vi "Parse Response Message.vi"(11 "message":string) -> (3 "response":T1 {"header"."response code" items=["NoError"=0, "FormErr"=1, "ServFail"=2, "NXDomain"=3, "NotImp"=4, "Refused"=5, "YXDomain"=6, "YXRRSet"=7, "NXRRSet"=8, "NotAuth"=9, "NotZone"=10, "DSOTYPENI"=11, "BADVERS/BADSIG"=16, "BADKEY"=17, "BADTIME"=18, "BADMODE"=19, "BADNAME"=20, "BADALG"=21, "BADTRUNC"=22, "BADCOOKIE"=23]; "header"."opcode" items=["Query"=0, "IQuery"=1, "Status"=2, "Notify"=4, "Update"=5, "DSO"=6]; "additional records"."class" items=["IN"=1, "CH"=3, "HS"=4]; "additional records"."type" items=["A"=1, "NS"=2, "MD"=3, "MF"=4, "CNAME"=5, "SOA"=6, "MB"=7, "MG"=8, "MR"=9, "NULL"=10, "WKS"=11, "PTR"=12, "HINFO"=13, "MINFO"=14, "MX"=15, "TXT"=16, "RP"=17, "AFSDB"=18, "X25"=19, "ISDN"=20, "RT"=21, "NSAP"=22, "NSAP-PTR"=23, "SIG"=24, "KEY"=25, "PX"=26, "GPOS"=27, "AAAA"=28, "LOC"=29, "NXT"=30, "EID"=31, "NIMLOC"=32, "SRV"=33, "ATMA"=34, "NAPTR"=35, "KX"=36, "CERT"=37, "A6"=38, "DNAME"=39, "SINK"=40, "OPT"=41, "APL"=42, "DS"=43, "SSHFP"=44, "IPSECKEY"=45, "RRSIG"=46, "NSEC"=47, "DNSKEY"=48, "DHCID"=49, "NSEC3"=50, "NSEC3PARAM"=51, "TLSA"=52, "SMIMEA"=53, "HIP"=55, "NINFO"=56, "RKEY"=57, "TALINK"=58, "CDS"=59, "CDNSKEY"=60, "OPENPGPKEY"=61, "CSYNC"=62, "ZONEMD"=63, "SVCB"=64, "HTTPS"=65, "SPF"=99, "UINFO"=100, "UID"=101, "GID"=102, "UNSPEC"=103, "NID"=104, "L32"=105, "L64"=106, "LP"=107, "EUI48"=108, "EUI64"=109, "URI"=256, "CAA"=257, "AVC"=258, "DOA"=259, "AMTRELAY"=260, "TA"=32768, "DLV"=32769]; "authority records"."class" items=["IN"=1, "CH"=3, "HS"=4]; "authority records"."type" items=["A"=1, "NS"=2, "MD"=3, "MF"=4, "CNAME"=5, "SOA"=6, "MB"=7, "MG"=8, "MR"=9, "NULL"=10, "WKS"=11, "PTR"=12, "HINFO"=13, "MINFO"=14, "MX"=15, "TXT"=16, "RP"=17, "AFSDB"=18, "X25"=19, "ISDN"=20, "RT"=21, "NSAP"=22, "NSAP-PTR"=23, "SIG"=24, "KEY"=25, "PX"=26, "GPOS"=27, "AAAA"=28, "LOC"=29, "NXT"=30, "EID"=31, "NIMLOC"=32, "SRV"=33, "ATMA"=34, "NAPTR"=35, "KX"=36, "CERT"=37, "A6"=38, "DNAME"=39, "SINK"=40, "OPT"=41, "APL"=42, "DS"=43, "SSHFP"=44, "IPSECKEY"=45, "RRSIG"=46, "NSEC"=47, "DNSKEY"=48, "DHCID"=49, "NSEC3"=50, "NSEC3PARAM"=51, "TLSA"=52, "SMIMEA"=53, "HIP"=55, "NINFO"=56, "RKEY"=57, "TALINK"=58, "CDS"=59, "CDNSKEY"=60, "OPENPGPKEY"=61, "CSYNC"=62, "ZONEMD"=63, "SVCB"=64, "HTTPS"=65, "SPF"=99, "UINFO"=100, "UID"=101, "GID"=102, "UNSPEC"=103, "NID"=104, "L32"=105, "L64"=106, "LP"=107, "EUI48"=108, "EUI64"=109, "URI"=256, "CAA"=257, "AVC"=258, "DOA"=259, "AMTRELAY"=260, "TA"=32768, "DLV"=32769]; "answers"."class" items=["IN"=1, "CH"=3, "HS"=4]; "answers"."type" items=["A"=1, "NS"=2, "MD"=3, "MF"=4, "CNAME"=5, "SOA"=6, "MB"=7, "MG"=8, "MR"=9, "NULL"=10, "WKS"=11, "PTR"=12, "HINFO"=13, "MINFO"=14, "MX"=15, "TXT"=16, "RP"=17, "AFSDB"=18, "X25"=19, "ISDN"=20, "RT"=21, "NSAP"=22, "NSAP-PTR"=23, "SIG"=24, "KEY"=25, "PX"=26, "GPOS"=27, "AAAA"=28, "LOC"=29, "NXT"=30, "EID"=31, "NIMLOC"=32, "SRV"=33, "ATMA"=34, "NAPTR"=35, "KX"=36, "CERT"=37, "A6"=38, "DNAME"=39, "SINK"=40, "OPT"=41, "APL"=42, "DS"=43, "SSHFP"=44, "IPSECKEY"=45, "RRSIG"=46, "NSEC"=47, "DNSKEY"=48, "DHCID"=49, "NSEC3"=50, "NSEC3PARAM"=51, "TLSA"=52, "SMIMEA"=53, "HIP"=55, "NINFO"=56, "RKEY"=57, "TALINK"=58, "CDS"=59, "CDNSKEY"=60, "OPENPGPKEY"=61, "CSYNC"=62, "ZONEMD"=63, "SVCB"=64, "HTTPS"=65, "SPF"=99, "UINFO"=100, "UID"=101, "GID"=102, "UNSPEC"=103, "NID"=104, "L32"=105, "L64"=106, "LP"=107, "EUI48"=108, "EUI64"=109, "URI"=256, "CAA"=257, "AVC"=258, "DOA"=259, "AMTRELAY"=260, "TA"=32768, "DLV"=32769]})   [LabVIEW 2015, in "PL DNS Client.lvlib"]
doc: "Parses DNS response <b>message</b>."
uses:
  PL DNS Client.lvlib
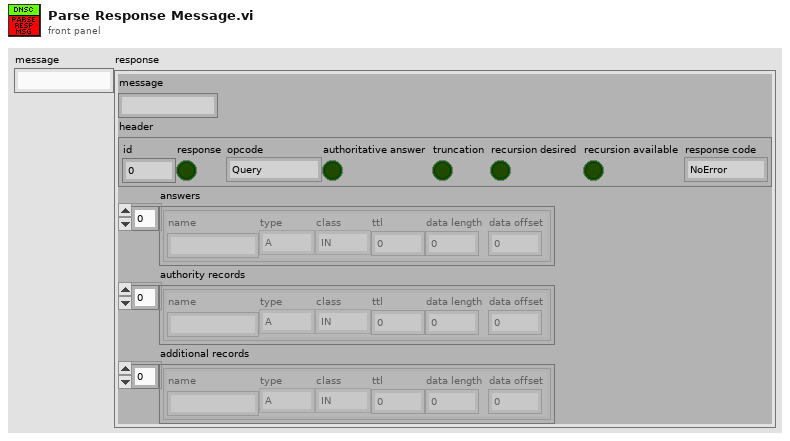
[diagram p1: front panel]
types:
  T1 = cluster{"message":string, "header":cluster{"id":u16, "response":bool, "opcode":u8, "authoritative answer":bool, "truncation":bool, "recursion desired":bool, "recursion available":bool, "response code":u16}, "answers":cluster{"name":string, "type":u16, "class":u16, "ttl":u32, "data length":u16, "data offset":u16}[], "authority records":cluster{"name":string, "type":u16, "class":u16, "ttl":u32, "data length":u16, "data offset":u16}[], "additional records":cluster{"name":string, "type":u16, "class":u16, "ttl":u32, "data length":u16, "data offset":u16}[]}
  T2 = cluster{"name":string, "type":u16, "class":u16, "ttl":u32, "data length":u16, "data offset":u16}
  T3 = cluster{cluster{"name":string, "type":u16, "class":u16, "ttl":u32, "data length":u16, "data offset":u16}[]}
  T4 = cluster{"name":string, "type":u16, "class":u16, "ttl":u32, "data length":u16, "data offset":u16}[]
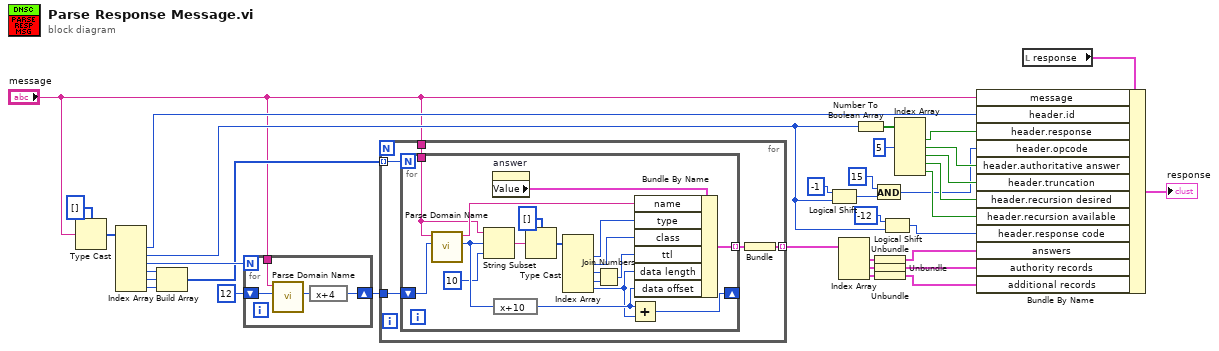
[diagram p0: block diagram]
diagram:
  n1 = Type Cast(type=u16[] [] ("array"), x="message") -> (*(type *) &x=w33:u16[])
  n2 = Index Array(array=w33) -> (element #1=w13:u16, element #2=w2:u16, element #3=w32:u16, element #4=w31:u16, element #5=w29:u16, element #6=w30:u16)  [unwired: 6 in]
  n3 = Build Array(w31, w29, w30) -> (w28:u16[])
  n4 = for {
    N: w32 -> [_]
    shift-right: [w36] -> w27
    shift-left: u16 12 -> [w38]
    tunnel: "message" -> [w35]
    n5 = call "Parse Domain Name.vi"("offset"=w38, "message"=w35) -> ("offset past domain name"=w37:u16)  [unwired: 8 in, 1 out]
    n6 = expression code="x+4"(w37) -> (w36:u16)
  }
  n7 = for {
    tunnel: w27 -> [w43]
    tunnel: "message" -> [w42]
    tunnel: w28 -> [w41] mode=indexing
    tunnel: [w39] -> w25 mode=indexing
    n8 = for {
      N: w41 -> [_]
      tunnel: w42 -> [w46]
      shift-right: [w60] -> _
      shift-left: w43 -> [w58]
      tunnel: [w61] -> w40 mode=indexing
      n9 = call "Parse Domain Name.vi"("offset"=w58, "message"=w46) -> ("offset past domain name"=w45:u16, "domain name"=w55:string)  [unwired: 8 in]
      n10 = String Subset(string=w46, offset (0)=w45, length (rest)=10 ("length")) -> (substring=w53:string)
      n11 = property on="answer" class="Clust (strict)"() -> ("Value"=w59:T2)  [unwired: 2 in, 2 out]
      n12 = expression code="x+10"(w45) -> (w56:u16)
      n13 = Type Cast(type=u16[] [] ("array"), x=w53) -> (*(type *) &x=w52:u16[])
      n14 = Index Array(array=w52) -> (element #1=w51:u16, element #2=w50:u16, element #3=w49:u16, element #4=w48:u16, element #5=w47:u16)  [unwired: 5 in]
      n15 = Join Numbers(hi=w49, lo=w48) -> ((hi.lo)=w57:u32)
      n16 = Add(x=w56, y=w47) -> (x+y=w60:u16)
      n17 = Bundle By Name(cluster=w59, "name"=w55, "type"=w51, "class"=w50, "ttl"=w57, "data length"=w47, "data offset"=w56) -> (w61:T2)
    }
    n18 = Bundle(w40) -> (w39:T3)  [unwired: 1 in]
  }
  n19 = Logical Shift(y=i16 -1, x=w2) -> (x << y=w4:u16)
  n20 = Index Array(array=w25) -> (element #1=w24:T3, element #2=w23:T3, element #3=w22:T3)  [unwired: 3 in]
  n21 = Number To Boolean Array(number=w2) -> (Boolean array=w18:bool[])
  n22 = And(x=u16 15, y=w4) -> (x .and. y?=w5:u16)
  n23 = Unbundle(w24) -> (w21:T4)
  n24 = Unbundle(w23) -> (w20:T4)
  n25 = Unbundle(w22) -> (w19:T4)
  n26 = Logical Shift(y=i16 -12, x=w2) -> (x << y=w16:u16)
  n27 = Index Array(array=w18, index #2=5 ("index")) -> (element #1=w12:bool, element #2=w10:bool, element #3=w9:bool, element #4=w8:bool, element #5=w7:bool)  [unwired: 4 in]
  n28 = local read "response"() -> (w14:T1)
  n29 = Bundle By Name(cluster=w14, "message"="message", "header.id"=w13, "header.response"=w12, "header.opcode"=w5, "header.authoritative answer"=w10, "header.truncation"=w9, "header.recursion desired"=w8, "header.recursion available"=w7, "header.response code"=w16, "answers"=w21, "authority records"=w20, "additional records"=w19) -> (→"response":T1)
